vi "GraphsQueue.vi"() -> ()   [LabVIEW 2019, in "Global.lvlib"]
uses:
  Global.lvlib
panel:
  in  "GraphQueue":i16
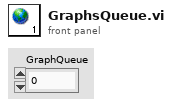
[diagram p1: front panel]
diagram:
